vi "Interface_Asset_Create DVR.vi"(8 "error in (no error)":errorcluster, 11 "AssetInterface in":refnum<class "Interface_Asset.lvclass">) -> (0 "error out":errorcluster, 3 "data value reference":refnum<data-value>)   [LabVIEW 2015, in "Interface_Asset.lvclass"]
uses:
  Interface_Asset.lvclass
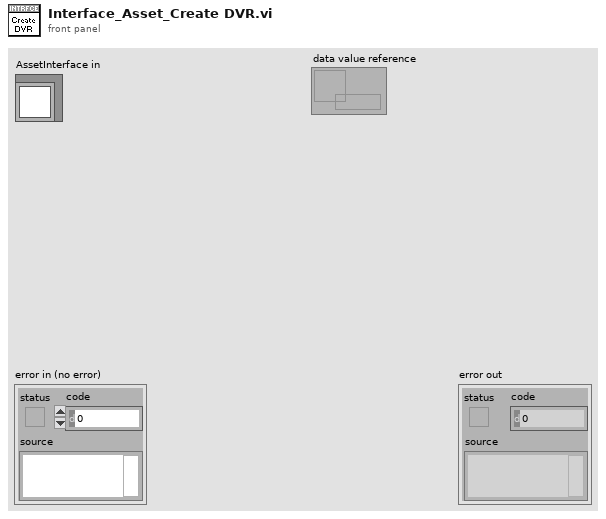
[diagram p1: front panel]
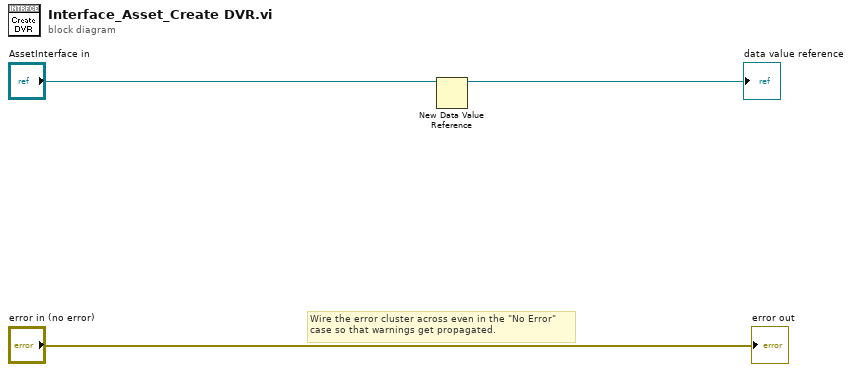
[diagram p0: block diagram]
diagram:
  # "Wire the error cluster across even in the \"No Error\"\ncase so that warnings get propagated."
  n1 = New Data Value Reference(data value="AssetInterface in") -> (data value reference=→"data value reference":refnum<data-value>)  [unwired: 1 in, 1 out]
  "error out" <- "error in (no error)"
